vi "Sample_Scan_Move_to_first_Pos.vi"(6 "semaphore":T1, 7 "use semaphore?":bool=TRUE, 8 "error in":errorcluster, 10 "Sample Scan Array In":i32[][](array[numeric]), 11 "ComPort":refnum<visa-resource-name>="COM11") -> (0 "error out":errorcluster, 1 "At first Pos?":bool, 2 "Sample Scan Array Out":i32[][](array[numeric]), 3 "VISA ressource out":refnum<visa-resource-name>, 4 "semaphore out":T1)   [LabVIEW 2018]
uses:
  MCode_LV_86/Set Parameter.ctl
  Surveillance/Pressure_Ch_1_2_Manipulator_Pos.vi
  Global_Next_Scan_Position.vi
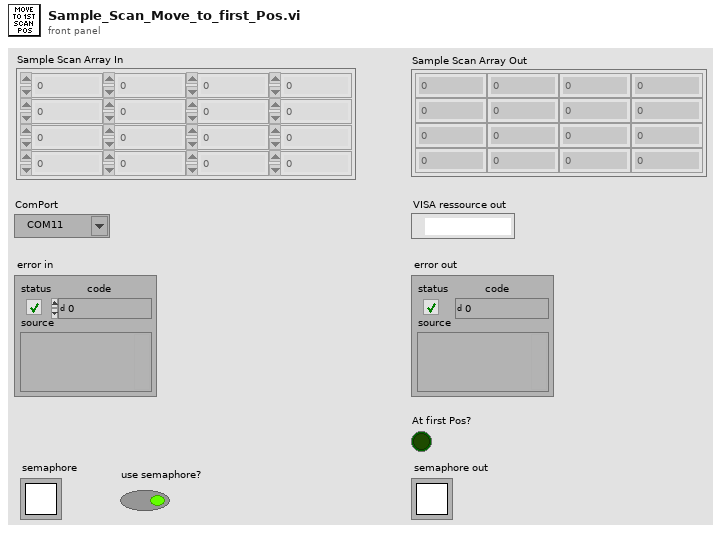
[diagram p1: front panel]
types:
  T1 = typedef "Semaphore RefNum" = refnum<k1>
  T2 = typedef "Set Parameter.ctl" = enum16{"Acceleration (A)", "Baud Rate (BD)", "Counter 1 (C1)", "Counter 2 (C2)", "Control C Software Reset (CE)", "Check Sum Enable (CK)", "Clock Mode (CM)", "Clock Mode Ratio (CR)", "Clock Mode Out Step Width (CW)", "Deceleration (D)", "Digital Filtering, Input 1 (D1)", "Digital Filtering, Input 2 (D2)", "Digital Filtering, Input 3 (D3)", "Digital Filtering, Input 4 (D4)", "Digital Filtering, Input 5 (D5)", "Digital Filtering, Input 9 (D9)", "Digital Filtering, Input 10 (D10)", "Digital Filtering, Input 11 (D11)", "Digital Filtering, Input 12 (D12)", "Deadband (DB)", "Decrement Variable (DC)", "Enable/Disable Drive (DE)", "Device Name (DN)", "End Program Execution (E)", "Encoder Function Enable (EE)", "Error Flag (EF)", "Encoder Lines (EL)", "Echo Mode (EM)", "Error Value (ER)", "Escape (ES)", "Execute Program at Address (EX)", "Firmware Version (VR)", "Hold (H)", "Hold Current (HC)", "Hold Current Delay Time (HI)", "Home to Encoder Index (HM)", "Home to Home Switch (HT)", "Increment Variable (IC)", "Initialize Parameters to NVM (IP)", "Input into Variable (IV)", "Jog Enable (JE)", "Limit Stop Mode (LM)", "Move Absolute (MA)", "Move Relative (MR)", "MicroStepping Select (MS)", "Motor Settling Delay Time (MT)", "Moving [Flag] (MV)", "Output 1 (O1)", "Output 2 (O2)", "Output 3 (O3)", "Output 4 (O4)", "Output 9 (O9)", "Output 10 (O10)", "Output 11 (O11)", "Output 12 (O12)", "Output High Byte (9-12) (OH)", "Output Low Byte (1-4) (OL)", "Output Total (1-4 and 9-12) (OT)", "Position (P)", "Position Maintenance (PM)", "Party Mode (PY)", "Register 1 (R1)", "Register 2 (R2)", "Register 3 (R3)", "Register 4 (R4)", "Reset Error(\\03)", "Run Current (RC)", "Stall Factor (SF)", "Slew (SL)", "Stall Mode Set (SM)", "Upgrade Firmware (UG)", "Velocity Initial (VI)", "Velocity Maximum (VM)", "Current1 (I1)", "Current2 (I2)", "Current3 (I3)", "Current4 (I4)", "Current5 (I5)", "Current6 (I6)", "Save (S)"}
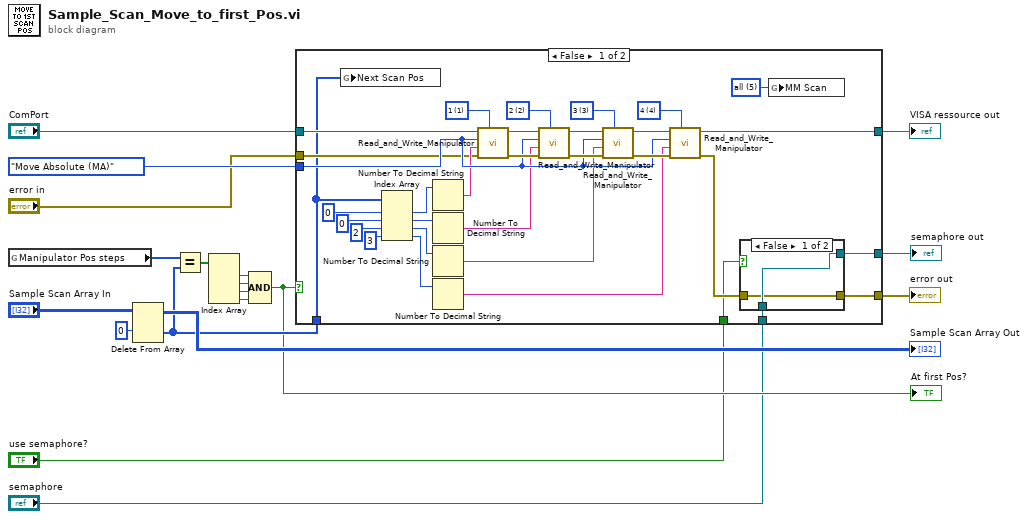
[diagram p0: block diagram]
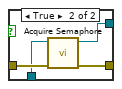
[diagram p2: hidden frame]
diagram:
  n1 = global read "Pressure_Ch_1_2_Manipulator_Pos.vi" "Manipulator Pos steps"() -> (w19:i32[])
  n2 = Delete From Array(array="Sample Scan Array In", index (row)=0) -> (deleted portion=w10:i32[], array with subset deleted=→"Sample Scan Array Out":i32[][])  [unwired: 2 in]
  n3 = Equal?(x=w19, y=w10) -> (x = y?=w18:bool[])
  n4 = Index Array(array=w18) -> (element #1=w17:bool, element #2=w16:bool, element #3=w15:bool, element #4=w14:bool)  [unwired: 4 in]
  n5 = Compound Arithmetic op=AND(w17, w16, w15, w14) -> (w4:bool)
  "At first Pos?" <- w4
  n6 = case shown="False" w4 {
    tunnel: w10 -> [w22 _]
    tunnel: "ComPort" -> [w42 w61]
    tunnel: Set_Parameter."Move Absolute (MA)" ("Command") -> [w41 _]
    tunnel: [w40 w61] -> w7
    tunnel: "error in" -> [w27 w60]
    tunnel: [w25 w60] -> w5
    tunnel: "semaphore" -> [w24 w59]
    tunnel: [w23 w59] -> w2
    tunnel: "use semaphore?" -> [w20 _]
    frame False {
      w21 = u16 5 items=["none", "1", "2", "3", "4", "all"] ("Motor 6")
      (unwired) 0 ("index")
      w52 = u16 4 items=["none", "1", "2", "3", "4", "all"] ("Motor")
      w51 = u16 3 items=["none", "1", "2", "3", "4", "all"] ("Motor")
      w50 = u16 2 items=["none", "1", "2", "3", "4", "all"] ("Motor")
      w49 = u16 1 items=["none", "1", "2", "3", "4", "all"] ("Motor")
      n7 = global write "Global_Next_Scan_Position.vi" "Next Scan Pos"(w22) -> ()
      n8 = Index Array(array=w22, index #1=0 ("index"), index #2=1 ("index"), index #3=2 ("index"), index #4=3 ("index")) -> (element #1=w35:i32, element #2=w33:i32, element #3=w31:i32, element #4=w30:i32)
      n9 = Number To Decimal String(number=w35) -> (decimal integer string=w34:string)  [unwired: 1 in]
      n10 = Number To Decimal String(number=w33) -> (decimal integer string=w32:string)  [unwired: 1 in]
      n11 = Number To Decimal String(number=w31) -> (decimal integer string=w29:string)  [unwired: 1 in]
      n12 = Number To Decimal String(number=w30) -> (decimal integer string=w28:string)  [unwired: 1 in]
      n13 = call "Read_and_Write_Manipulator.vi"("Motor"=w49, "error in (no error)"=w27, "Value"=w34, "Command"=w41, "VISA resource name"=w42) -> ("error out"=w43:errorcluster, "VISA ressource out"=w46:refnum<visa-resource-name>)  [unwired: 2 in, 3 out]
      n14 = call "Read_and_Write_Manipulator.vi"("Motor"=w50, "error in (no error)"=w43, "Value"=w32, "Command"=w41, "VISA resource name"=w46) -> ("error out"=w44:errorcluster, "VISA ressource out"=w47:refnum<visa-resource-name>)  [unwired: 2 in, 3 out]
      n15 = call "Read_and_Write_Manipulator.vi"("Motor"=w51, "error in (no error)"=w44, "Value"=w29, "Command"=w41, "VISA resource name"=w47) -> ("error out"=w45:errorcluster, "VISA ressource out"=w48:refnum<visa-resource-name>)  [unwired: 2 in, 3 out]
      n16 = call "Read_and_Write_Manipulator.vi"("Motor"=w52, "error in (no error)"=w45, "Value"=w28, "Command"=w41, "VISA resource name"=w48) -> ("error out"=w26:errorcluster, "VISA ressource out"=w40:refnum<visa-resource-name>)  [unwired: 2 in, 3 out]
      n17 = case shown="False" w20 {
        tunnel: w26 -> [w53 w58]
        tunnel: [w53 w57] -> w25
        tunnel: w24 -> [w54 w56]
        tunnel: [w54 w55] -> w23
        frame False {
        }
        frame True {
          n18 = call <vilib>:"Acquire Semaphore.vi"("error in (no error)"=w58, "semaphore"=w56) -> ("error out"=w57:errorcluster, "semaphore out"=w55:T1)  [unwired: 3 in, 1 out]
        }
      }
      n19 = global write "Global_Next_Scan_Position.vi" "MM Scan"(w21) -> ()
    }
    frame True {
    }
  }
  "VISA ressource out" <- w7
  "error out" <- w5
  "semaphore out" <- w2
